vi "test broken tool.vi"(8 "error in (no error)":errorcluster) -> (0 "error out":errorcluster, 3 "body":string)   [LabVIEW 2025, in "MCP Server tests.lvlib"]
uses:
  MCP Server tests.lvlib
  <vilib>/addons/_JKI Toolkits/Caraya/classes/Test/Test.lvclass
  <vilib>/addons/_JKI Toolkits/Caraya/classes/Assert/Assert.lvclass
  <vilib>/JDP Science/JSONtext/JSONtext.lvlib
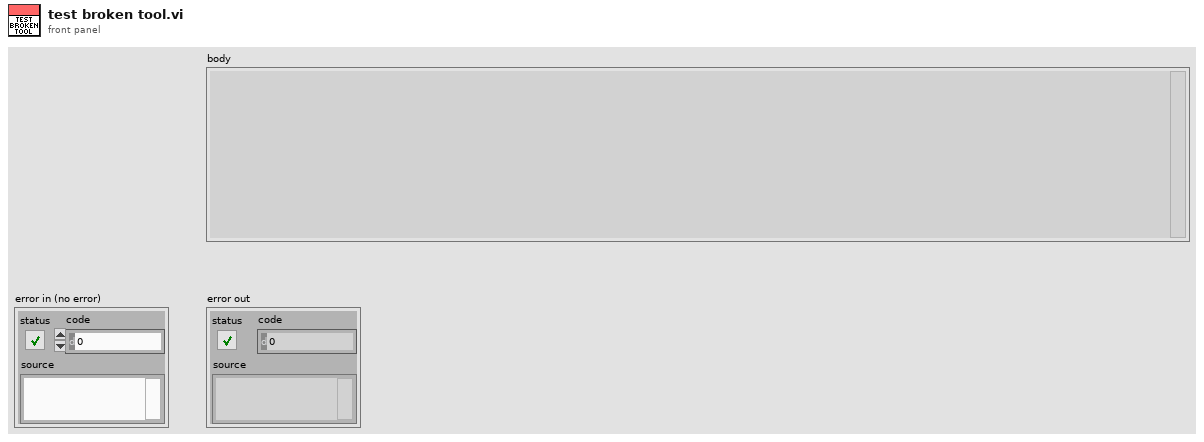
[diagram p1: front panel]
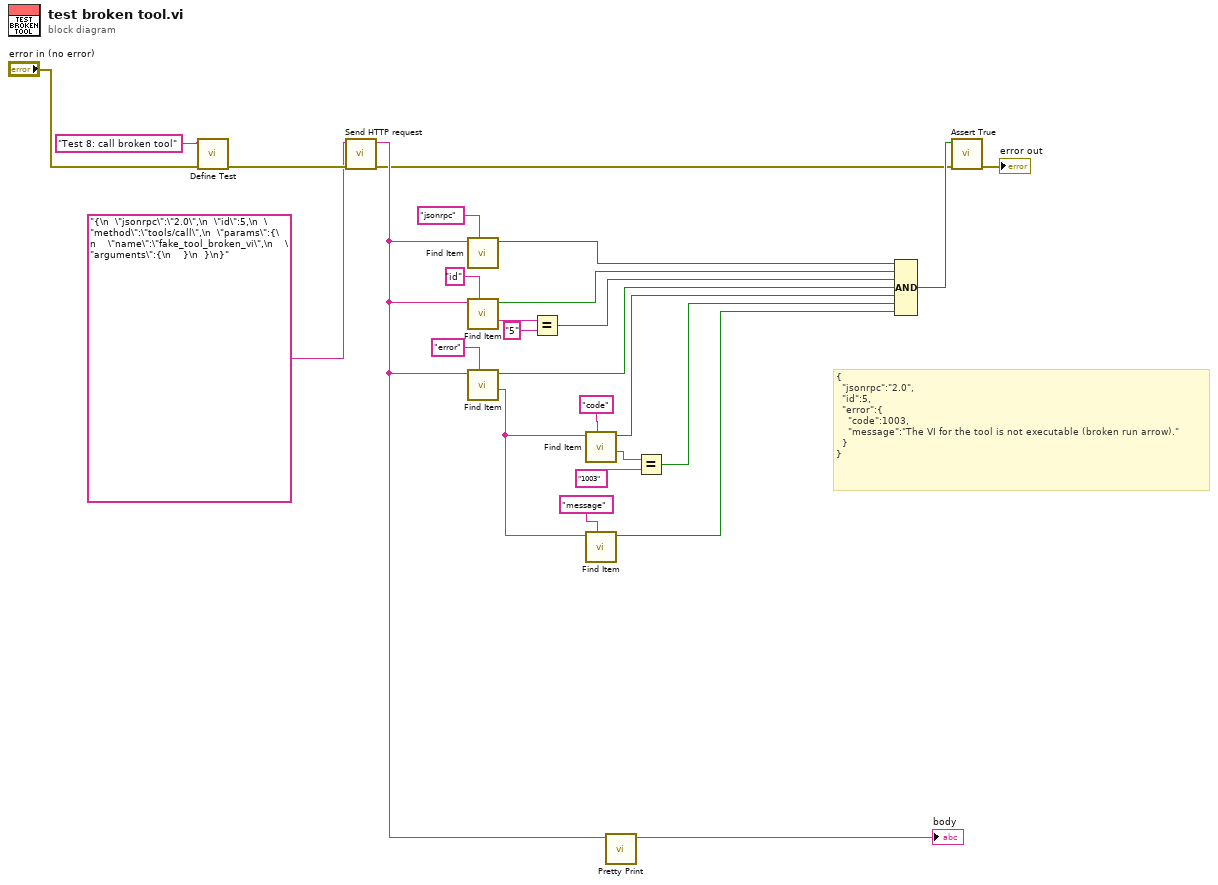
[diagram p0: block diagram]
diagram:
  # "{\n  \"jsonrpc\":\"2.0\",\n  \"id\":5,\n  \"error\":{\n    \"code\":1003,\n    \"message\":\"The VI for the tool is not executable (broken run arrow).\"\n  }\n}"
  n1 = call <vilib>:"Define Test.vi"("error in (no error)"="error in (no error)", "Label (VI Title)"="Test 8: call broken tool") -> ("error out"=w13:errorcluster)  [unwired: 8 in, 1 out]
  n2 = call "Send HTTP request.vi"("error in (no error)"=w13, "request"="{\n  \"jsonrpc\":\"2.0\",\n  \"id\":5,\n  \"method\":\"tools/call\",\n  \"params\":{\n    \"name\":\"fake_tool_broken_vi\",\n    \"arguments\":{\n    }\n  }\n}" ("buffer")) -> ("error out"=w14:errorcluster, "response"=w25:string)  [unwired: 7 in, 1 out]
  n3 = call <vilib>:"Find Item.vi"("$Path or Item Name"="jsonrpc", "JSON"=w25) -> ("Found"=w19:bool)  [unwired: 6 in, 3 out]
  n4 = call <vilib>:"Find Item.vi"("$Path or Item Name"="id", "JSON"=w25) -> ("<JSON>"=w17:string, "Found"=w20:bool)  [unwired: 6 in, 2 out]
  n5 = call <vilib>:"Find Item.vi"("$Path or Item Name"="error", "JSON"=w25) -> ("<JSON>"=w2:string, "Found"=w24:bool)  [unwired: 6 in, 2 out]
  n6 = Equal?(x=w17, y="5") -> (x = y?=w21:bool)
  n7 = call <vilib>:"Find Item.vi"("$Path or Item Name"="code", "JSON"=w2) -> ("<JSON>"=w6:string, "Found"=w7:bool)  [unwired: 6 in, 2 out]
  n8 = call <vilib>:"Find Item.vi"("$Path or Item Name"="message", "JSON"=w2) -> ("Found"=w1:bool)  [unwired: 6 in, 3 out]
  n9 = call <vilib>:"Pretty Print.vi"("JSON"=w25) -> ("<JSON>"=→"body":string)  [unwired: 8 in, 2 out]
  n10 = Equal?(x=w6, y="1003") -> (x = y?=w4:bool)
  n11 = Compound Arithmetic op=AND(w19, w20, w21, w24, w7, w4, w1) -> (w22:bool)
  n12 = call <vilib>:"Assert True.vi"("error in (no error)"=w14, "True?"=w22) -> ("error out"=→"error out":errorcluster)  [unwired: 8 in, 1 out]
